vi "Asyn Rx Ch Read.vi"(6 "pReturned":u32, 8 "pBuffer":u8[](array[numeric]), 9 "Length":u32, 10 "Channel":u8, 11 "devId":i32) -> (0 "pBuffer out":u8[](array[numeric]), 1 "devId out":i32, 3 "function return":i32, 4 "pReturned out":u32)   [LabVIEW 2013, in "CHR34XXX.lvlib"]
doc: "DLL BOOL __stdcall CHR34XXX_Asyn_RxCh_FIFOState(IN int devId,IN BYTE Channel,OUT DWORD *pState); DLL BOOL __stdcall CHR34XXX_Asyn_RxCh_FIFOCount(IN int devId,IN BYTE Channel,OUT DWORD *pCount); DLL BOOL __stdcall CHR34XXX_Asyn_RxCh_Read(IN int devId,IN BYTE Channel,IN DWORD Length,OUT BYTE *pBuffer,OUT DWORD *pReturned);"
uses:
  CHR34XXX.lvlib
  CHR34XXX.dll
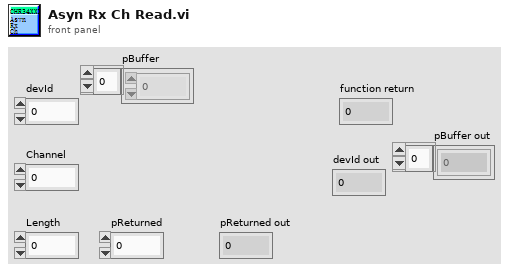
[diagram p1: front panel]
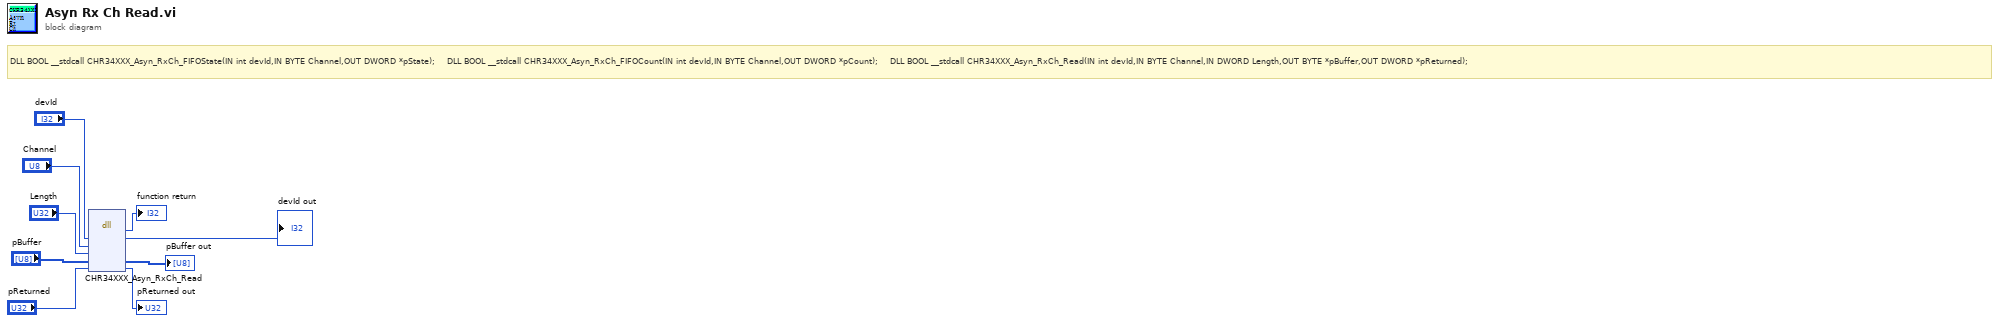
[diagram p0: block diagram]
diagram:
  # "DLL BOOL __stdcall CHR34XXX_Asyn_RxCh_FIFOState(IN int devId,IN BYTE Channel,OUT DWORD *pState);    DLL BOOL __stdcall CHR34XXX_Asyn_RxCh_FIFOCount(IN int devId,IN BYTE Channel,OUT DWORD *pCount);    DLL BOOL __stdcall CHR34XXX_Asyn_RxCh_Read(IN int devId,IN BYTE Channel,IN DWORD Length,OUT BYTE *pBuffer,OUT DWORD *pReturned);"
  n1 = dll-call lib="C:/Users/dy/Desktop/CHR34XXX_lv/lv_lib/CHR34XXX.*" fn="CHR34XXX_Asyn_RxCh_Read"("devId"="devId", "Channel"="Channel", "Length"="Length", "pBuffer"="pBuffer", "pReturned"="pReturned") -> ("返回类型"=→"function return":i32, "devId"=→"devId out":i32, "pBuffer"=→"pBuffer out":u8[], "pReturned"=→"pReturned out":u32)  [unwired: 5 in, 2 out]
